vi "FilterRoomEvents.vi"(8 "error in":errorcluster, 9 "Filter 3":T1={"Filter"=enum."Room Number", "From"=timestamp(0 s since 1904-01-01), "To"=timestamp(0 s since 1904-01-01), "Filter Text"="", "RoomNumFlags"={"Flag State"=[1, 3, 5, 7]}, "BedVacant"=FALSE, "Enable Filter"=FALSE}, 10 "Filter 2":T1={"Filter"=enum."Room Number", "From"=timestamp(0 s since 1904-01-01), "To"=timestamp(0 s since 1904-01-01), "Filter Text"="", "RoomNumFlags"={"Flag State"=[1, 3, 5, 7]}, "BedVacant"=FALSE, "Enable Filter"=FALSE}, 11 "Filter 1":T1={"Filter"=enum."Room Number", "From"=timestamp(0 s since 1904-01-01), "To"=timestamp(0 s since 1904-01-01), "Filter Text"="", "RoomNumFlags"={"Flag State"=[1, 3, 5, 7]}, "BedVacant"=FALSE, "Enable Filter"=FALSE}) -> (0 "error out":errorcluster, 1 "EventTimeArray":timestamp[](array[timestamp]), 2 "RoomArray":refnum<class "Room.lvclass">[](array[class]))   [LabVIEW 2015, in "DatabaseApi.lvlib"]
uses:
  DatabaseApi.lvlib
  TypeDef/Room/RoomFilter.ctl
  TypeDef/Room/RoomTableFilterRing.ctl
  LVClasses/Flags/ColorFlags.ctl
  LVClasses/Room/Room.lvclass
  LVClasses/Flags/Flags.lvclass
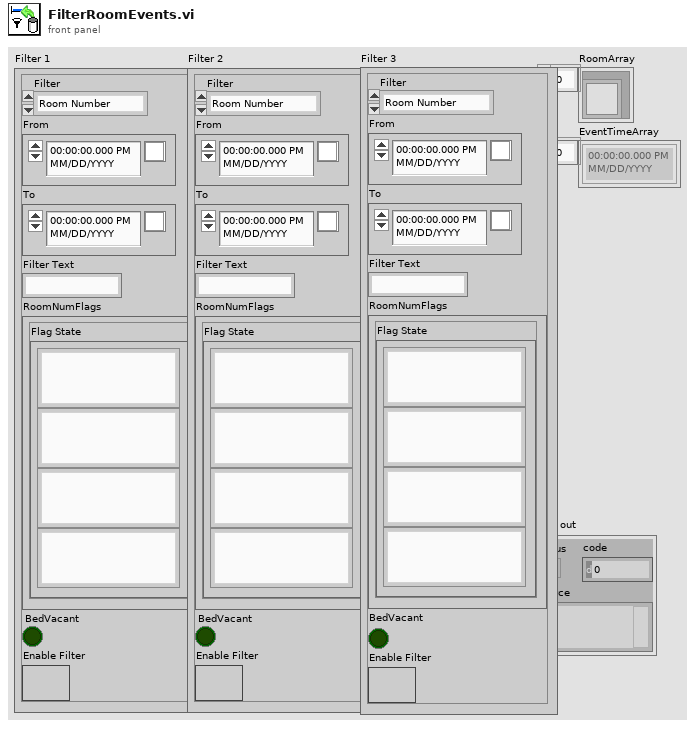
[diagram p1: front panel]
types:
  T1 = typedef "DatabaseApi.lvlib/RoomFilter.ctl" = cluster{"Filter":T2, "From":timestamp, "To":timestamp, "Filter Text":string, "RoomNumFlags":T3, "BedVacant":bool, "Enable Filter":bool}
  T2 = typedef "DatabaseApi.lvlib/RoomTableFilterRing.ctl" = enum16{"Room Number", "Event Time", "Flags", "Bed Vacant", "In Room Personnel"}
  T3 = typedef "Flags.lvclass/ColorFlags.ctl" = cluster{"Flag State":u8[]}
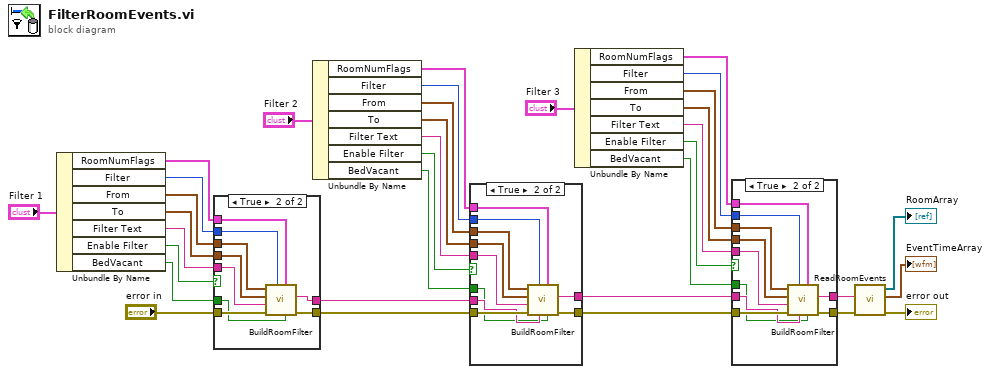
[diagram p0: block diagram]
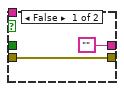
[diagram p4: hidden frame]
diagram:
  n1 = Unbundle By Name("Filter 1") -> ("RoomNumFlags"=w19:T3, "Filter"=w31:T2, "From"=w30:timestamp, "To"=w29:timestamp, "Filter Text"=w28:string, "Enable Filter"=w27:bool, "BedVacant"=w14:bool)
  n2 = case shown="True" w27 {
    tunnel: "error in" -> [w36 w45]
    tunnel: [w36 w44] -> w32
    tunnel: ["" w43] -> w21
    tunnel: w31 -> [_ w42]
    tunnel: w30 -> [_ w41]
    tunnel: w29 -> [_ w40]
    tunnel: w28 -> [_ w39]
    tunnel: w19 -> [_ w38]
    tunnel: w14 -> [_ w37]
    frame False {
    }
    frame True {
      n3 = call "BuildRoomFilter.vi"("BedVacant"=w37, "RoomNumFlags"=w38, "Filter"=w42, "error in"=w45, "Filter Text"=w39, "To"=w40, "From"=w41) -> ("error out"=w44:errorcluster, "condition"=w43:string)  [unwired: 3 in]
    }
  }
  n4 = Unbundle By Name("Filter 2") -> ("RoomNumFlags"=w17:T3, "Filter"=w26:T2, "From"=w25:timestamp, "To"=w24:timestamp, "Filter Text"=w23:string, "Enable Filter"=w22:bool, "BedVacant"=w13:bool)
  n5 = case shown="True" w22 {
    tunnel: w32 -> [w47 w57]
    tunnel: [w47 w56] -> w8
    tunnel: [w46 w55] -> w9
    tunnel: w26 -> [_ w54]
    tunnel: w25 -> [_ w53]
    tunnel: w24 -> [_ w52]
    tunnel: w23 -> [_ w51]
    tunnel: w21 -> [w46 w50]
    tunnel: w17 -> [_ w49]
    tunnel: w13 -> [_ w48]
    frame False {
    }
    frame True {
      n6 = call "BuildRoomFilter.vi"("BedVacant"=w48, "RoomNumFlags"=w49, "InputCondition"=w50, "Filter"=w54, "error in"=w57, "Filter Text"=w51, "To"=w52, "From"=w53) -> ("error out"=w56:errorcluster, "condition"=w55:string)  [unwired: 2 in]
    }
  }
  n7 = Unbundle By Name("Filter 3") -> ("RoomNumFlags"=w2:T3, "Filter"=w3:T2, "From"=w4:timestamp, "To"=w5:timestamp, "Filter Text"=w6:string, "Enable Filter"=w7:bool, "BedVacant"=w10:bool)
  n8 = case shown="True" w7 {
    tunnel: w8 -> [w59 w69]
    tunnel: [w59 w68] -> w12
    tunnel: [w58 w67] -> w11
    tunnel: w3 -> [_ w66]
    tunnel: w4 -> [_ w65]
    tunnel: w5 -> [_ w64]
    tunnel: w6 -> [_ w63]
    tunnel: w9 -> [w58 w62]
    tunnel: w2 -> [_ w61]
    tunnel: w10 -> [_ w60]
    frame False {
    }
    frame True {
      n9 = call "BuildRoomFilter.vi"("BedVacant"=w60, "RoomNumFlags"=w61, "InputCondition"=w62, "Filter"=w66, "error in"=w69, "Filter Text"=w63, "To"=w64, "From"=w65) -> ("error out"=w68:errorcluster, "condition"=w67:string)  [unwired: 2 in]
    }
  }
  n10 = call "ReadRoomEvents.vi"("error in"=w12, "condition"=w11) -> ("error out"=→"error out":errorcluster, "EventTimeArray"=→"EventTimeArray":timestamp[], "RoomArray"=→"RoomArray":refnum<class "Room.lvclass">[])  [unwired: 7 in]
